vi "Default Settings.vi"(8 "error in (no error)":errorcluster, 11 "Sensor Dispense in":refnum<class "Sensor Dispense.lvclass">) -> (0 "error out":errorcluster, 3 "Sensor Dispense out":refnum<class "Sensor Dispense.lvclass">)   [LabVIEW 2020, in "Sensor Dispense.lvclass"]
uses:
  Projects/Sensor Dispense.lvclass
  C:/Users/hep/Documents/UCSB-Gantry-2022/Classes/Routine/Dispense/Dispense.lvclass
  Projects/Sensor Dispense.lvclass/Sensor Dispense.ctl
  Dispense.lvclass/Dispense.ctl
  Write Tip Height.vi
  Dispense.lvclass
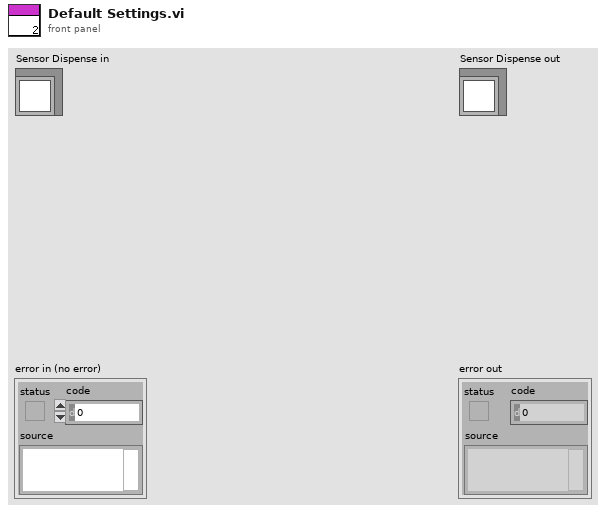
[diagram p1: front panel]
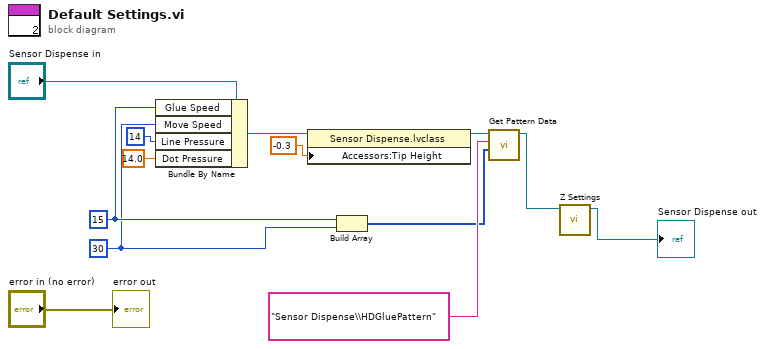
[diagram p0: block diagram]
diagram:
  w4 = 30
  w5 = 15
  n1 = Bundle By Name(cluster="Sensor Dispense in", "Glue Speed"=w5, "Move Speed"=w4, "Line Pressure"=14, "Dot Pressure"=14.0) -> (w11:refnum<class "Sensor Dispense.lvclass">)
  n2 = property class="Sensor Dispense.lvclass"(reference=w11, "Accessors:Tip Height"=-0.3) -> (reference out=w7:refnum<class "Sensor Dispense.lvclass">)  [unwired: 1 in, 1 out]
  n3 = Build Array(w5, w4) -> (w3:i32[])
  n4 = call "Get Pattern Data.vi"("File Name"=w3, "Folder Name"="Sensor Dispense\\HDGluePattern", "Dispense.lvclass"=w7) -> ("Dispense Out"=w2:refnum<class "Sensor Dispense.lvclass">)  [unwired: 8 in]
  n5 = call-dynamic "Z Settings.vi"("Dispense in"=w2) -> ("Dispense out"=→"Sensor Dispense out":refnum<class "Sensor Dispense.lvclass">)  [unwired: 9 in, 1 out]
  "error out" <- "error in (no error)"
